vi "FrecAmpGEN.vi"(8 "error in (no error)":errorcluster, 9 "Frec (Hz)":dbl, 10 "Amplitud (Vrms)":dbl) -> (0 "error out":errorcluster, 3 "DS360 out":refnum<class "DS360.lvclass">)   [LabVIEW 2019, in "DS360.lvclass"]
uses:
  DS360.lvclass
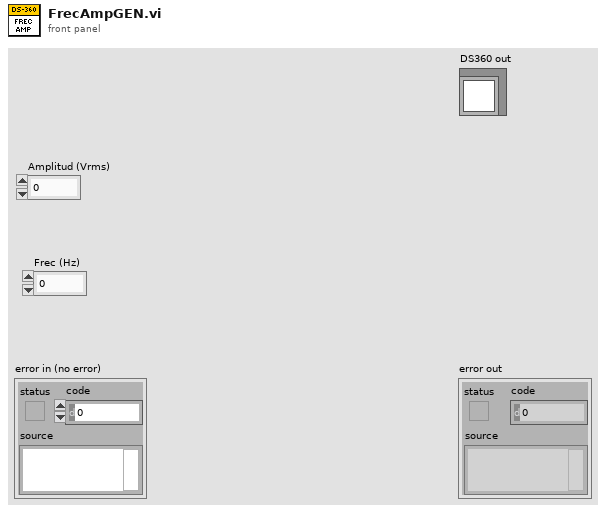
[diagram p1: front panel]
types:
  T1 = cluster{"error":bool, "code":i32, "source":string}
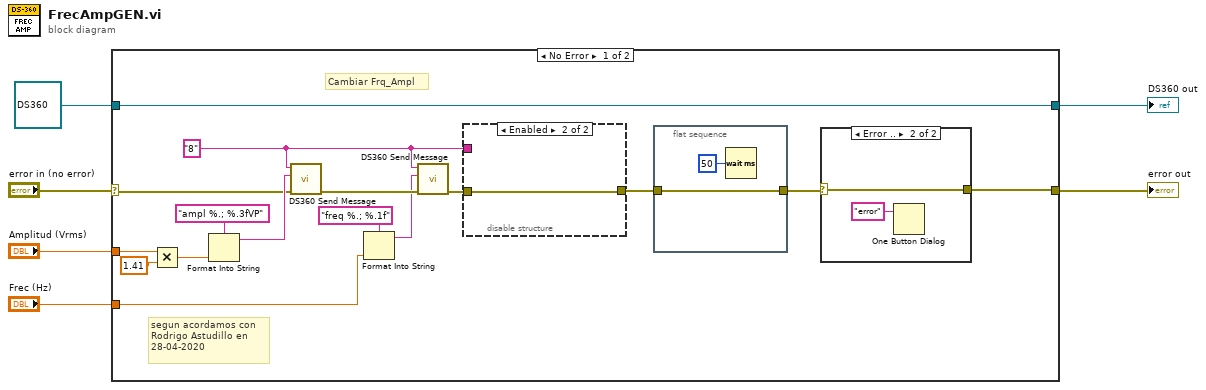
[diagram p0: block diagram]
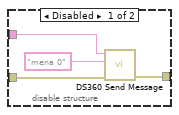
[diagram p3: hidden frame]
diagram:
  n1 = case shown="No Error" "error in (no error)" {
    selector: "error in (no error)" -> [w14 w34]
    tunnel: [w7 w34] -> w5
    tunnel: [w22 w33] -> w3
    tunnel: refnum<class "DS360.lvclass"> refnum ("DS360 in") -> [w22 w33]
    tunnel: "Amplitud (Vrms)" -> [w12 _]
    tunnel: "Frec (Hz)" -> [w13 _]
    frame No Error {
      w15 = "8" ("write buffer")
      # "segun acordamos con\nRodrigo Astudillo en\n28-04-2020"
      # "Cambiar Frq_Ampl"
      n2 = Multiply(x=w12, y=1.41) -> (x*y=w10:dbl)
      n3 = Format Into String(format string="ampl %.; %.3fVP" ("write buffer"), w10) -> (resulting string=w18:string)  [unwired: 2 in, 1 out]
      n4 = call <instrlib>:"DS360 Send Message.vi"("address string"=w15, "write buffer"=w18, "error in"=w14) -> ("error out"=w21:T1)  [unwired: 3 in, 3 out]
      n5 = Format Into String(format string="freq %.; %.1f" ("write buffer"), w13) -> (resulting string=w16:string)  [unwired: 2 in, 1 out]
      n6 = call <instrlib>:"DS360 Send Message.vi"("address string"=w15, "write buffer"=w16, "error in"=w21) -> ("error out"=w20:T1)  [unwired: 3 in, 3 out]
      n7 = disable-structure shown="Enabled" {
        disable-tunnel: w20 -> [w30 w32]
        disable-tunnel: w15 -> [w29 _]
        disable-tunnel: [w28 w32] -> w9
        frame Disabled {
          n8 = call <instrlib>:"DS360 Send Message.vi"("address string"=w29, "write buffer"="mena 0", "error in"=w30) -> ("error out"=w28:T1)  [unwired: 3 in, 3 out]
        }
        frame Enabled {
        }
      }
      n9 = flat-sequence {
        tunnel: w9 -> [w26]
        tunnel: [w26] -> w8
        frame #0 {
          n10 = Wait (ms)(milliseconds to wait=u32 50) -> ()  [unwired: 1 out]
        }
      }
      n11 = case shown="Error .." w8 {
        selector: w8 -> [w23 w25]
        tunnel: [w23 w25] -> w7
        frame No Error {
        }
        frame Error {
          n12 = One Button Dialog(message="error") -> ()  [unwired: 1 in, 1 out]
        }
      }
    }
    frame Error {
    }
  }
  "error out" <- w5
  "DS360 out" <- w3
